vi "Compression_Simulation_Get GAINs.vi"(6 "Adjusting Factor":dbl, 9 "Max Linear Range (dBm)":dbl, 10 "Expected DUT Gain (dB)":dbl, 11 "PINs in":dbl[](array[numeric])) -> (2 "Linear Gain":dbl, 3 "GAINs out":dbl[](array[numeric]))   [LabVIEW 2023]
uses:
  <vilib>/Analysis/baseanly.llb/Mean (DBL).vi
  <vilib>/Analysis/NI_AALBase.lvlib
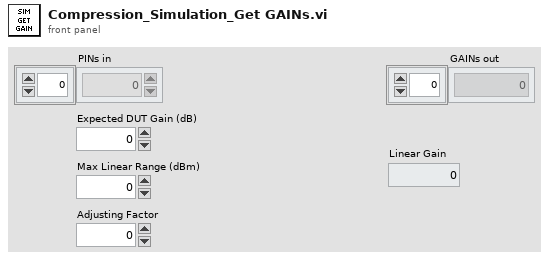
[diagram p1: front panel]
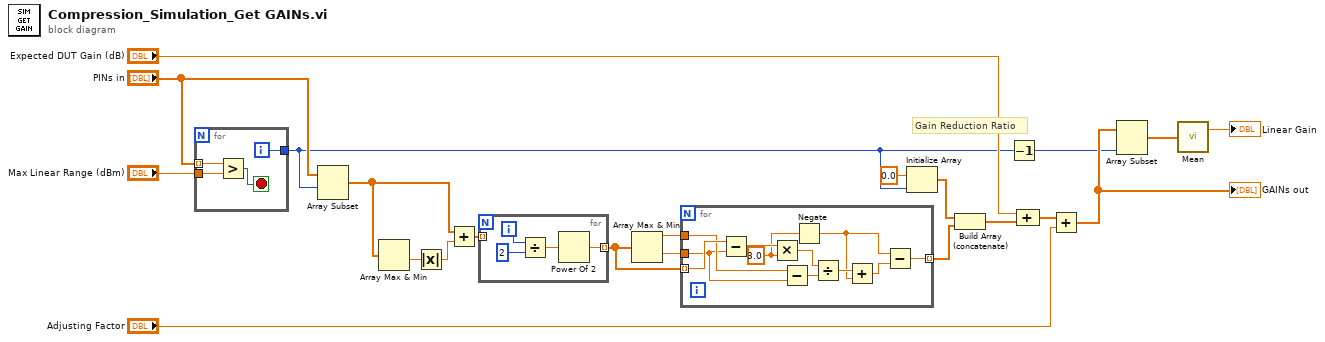
[diagram p0: block diagram]
diagram:
  # "Gain Reduction Ratio"
  n1 = for {
    tunnel: "PINs in" -> [w24] mode=indexing
    tunnel: "Max Linear Range (dBm)" -> [w23]
    tunnel: [w22] -> w3
    i -> [w22]
    stop <- w25 stop-if-true
    n2 = Greater?(x=w24, y=w23) -> (0:w25:bool)
  }
  n3 = Array Subset(array="PINs in", index=w3) -> (w14:dbl[])  [unwired: 1 in]
  n4 = Array Max & Min(array=w14) -> (min value=w15:dbl)  [unwired: 3 out]
  n5 = Absolute Value(x=w15) -> (abs(x)=w16:dbl)
  n6 = Add(x=w14, y=w16) -> (x+y=w13:dbl[])
  n7 = for {
    tunnel: [w29] -> w20 mode=indexing
    tunnel: w13 -> [_] mode=indexing
    i -> [w28]
    n8 = Divide(x=w28, y=2) -> (x/y=w27:dbl)
    n9 = Power Of 2(x=w27) -> (2^x=w29:dbl)
  }
  n10 = Array Max & Min(array=w20) -> (max value=w7:dbl, min value=w8:dbl)  [unwired: 2 out]
  n11 = for {
    tunnel: w7 -> [w39]
    tunnel: w20 -> [w40] mode=indexing
    tunnel: [w32] -> w11 mode=indexing
    tunnel: w8 -> [w38]
    w33 = 3.0 ("y")
    n12 = Subtract(x=w40, y=w38) -> (x-y=w36:dbl)
    n13 = Multiply(x=w36, y=w33) -> (x*y=w35:dbl)
    n14 = Subtract(x=w39, y=w38) -> (x-y=w37:dbl)
    n15 = Negate(x=w33) -> (-x=w31:dbl)
    n16 = Divide(x=w35, y=w37) -> (x/y=w34:dbl)
    n17 = Add(x=w34, y=w31) -> (x+y=w30:dbl)
    n18 = Subtract(x=w31, y=w30) -> (x-y=w32:dbl)
  }
  n19 = Initialize Array(0.0 ("element"), w3) -> (w10:dbl[])
  n20 = Build Array (concatenate)(w10, w11) -> (w17:dbl[])
  n21 = Decrement(x=w3) -> (x-1=w2:i32)
  n22 = Compound Arithmetic op=ADD("Expected DUT Gain (dB)", w17) -> (w19:dbl[])
  n23 = Add(x=w19, y="Adjusting Factor") -> (x+y=w4:dbl[])
  "GAINs out" <- w4
  n24 = Array Subset(array=w4, length=w2) -> (w5:dbl[])  [unwired: 1 in]
  n25 = call-poly <vilib>:"Mean.vi"("X"=w5) -> ("mean"=→"Linear Gain":dbl)  [unwired: 1 out]
